vi "configureAcquisition.vi"(6 "imagePaths":path[](array[path]), 7 "saveImages?":bool, 8 "error in (no error)":errorcluster, 9 "number of Images":i32, 10 "CameraSettings":refnum<class "CamaraSettings.lvclass">, 11 "Camera in":refnum<class "Camera.lvclass">) -> (0 "error out":errorcluster, 3 "Camera out":refnum<class "Camera.lvclass">)   [LabVIEW 2009, in "Hardware.lvlib" / "Channels.lvlib" / "Camera.lvclass"]
uses:
  Camera.lvclass
  Tools/CameraSettings/CamaraSettings.lvclass
  Camera.lvclass/Camera.ctl
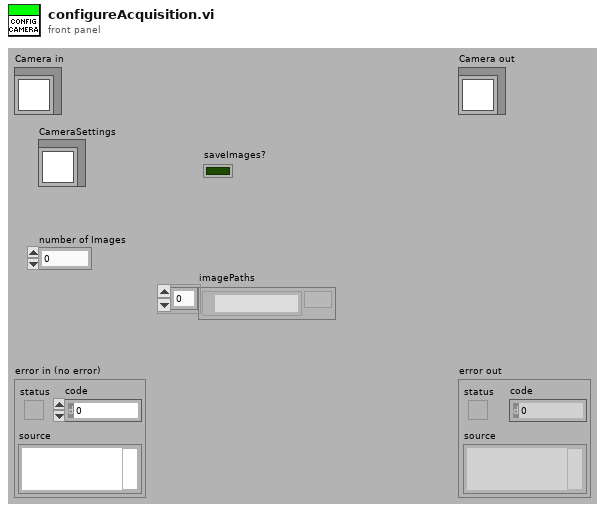
[diagram p1: front panel]
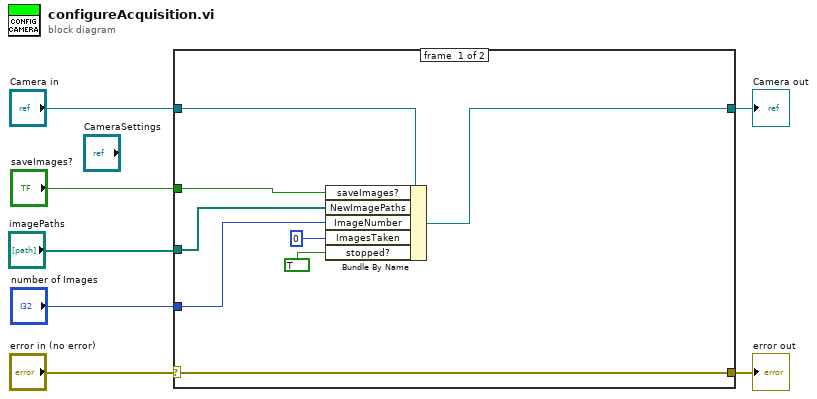
[diagram p0: block diagram]
diagram:
  n1 = case shown="No Error" "error in (no error)" {
    selector: "error in (no error)" -> [w15 w17]
    tunnel: [w15 w17] -> w6
    tunnel: [w12 w16] -> w4
    tunnel: "Camera in" -> [w13 w16]
    tunnel: "saveImages?" -> [w14 _]
    tunnel: "imagePaths" -> [w11 _]
    tunnel: "number of Images" -> [w10 _]
    frame #0 {
      n2 = Bundle By Name(cluster=w13, "saveImages?"=w14, "NewImagePaths"=w11, "ImageNumber"=w10, "ImagesTaken"=0, "stopped?"=TRUE) -> (w12:refnum<class "Camera.lvclass">)
    }
    frame #1 {
    }
  }
  "error out" <- w6
  "Camera out" <- w4
